vi "Handling calc param full_ext.vi"(0 "PV":dbl step=0.009999999776482582, 1 "SOURCE":u32=1 max=2 step=1, 2 "SOURCE_ALLOW":bool, 3 "PV2":dbl step=0.009999999776482582, 4 "control":T2={"GAIN"=1.0, "OFFSET"=0.0, "TIME_CONST"=100.0, "MINOFFSET"=2.0, "PVMIN"=0.0, "MINACC"=0.0, "LL"=1.0, "L"=2.0, "H"=8.0, "HH"=9.0, "MAXACC"=9.5, "PVMAX"=10.0, "MAXOFFSET"=2.0, "D"=0.5, "VMAX"=0.0, "TOUT"=1.0, "APERTURE"=0.0} {"APERTURE" min=-100000.0 max=100000.0 step=0.0010000000474974513; "TOUT" min=0.0 max=100000.0 step=1.0; "D" min=-100000.0 max=100000.0 step=0.0010000000474974513; "MAXOFFSET" min=0.0 max=50.0 step=0.0010000000474974513; "PVMAX" min=-100000.0 max=100000.0 step=0.0010000000474974513; "MAXACC" min=-100000.0 max=100000.0 step=0.0010000000474974513; "HH" min=-100000.0 max=100000.0 step=0.0010000000474974513; "H" min=-100000.0 max=100000.0 step=0.0010000000474974513; "L" min=-100000.0 max=100000.0 step=0.0010000000474974513; "LL" min=-100000.0 max=100000.0 step=0.0010000000474974513; "MINACC" min=-100000.0 max=100000.0 step=0.0010000000474974513; "PVMIN" min=-100000.0 max=100000.0 step=0.0010000000474974513; "MINOFFSET" min=0.0 max=50.0 step=0.0010000000474974513; "TIME_CONST" min=1.0 max=100000.0 step=1.0; "OFFSET" min=-100000.0 max=100000.0 step=0.0010000000474974513; "GAIN" min=0.0010000000474974513 max=1000.0 step=0.0010000000474974513}, 6 "initialise":bool, 7 "Sensor handling full reg old":T1, 8 "code":i32) -> (13 "Sensor handling full reg":T1, 14 "PVOUT":dbl format="%#_3g", 15 "SOURCEOUT":u32=1 max=2 step=1, 16 "STATE":T3, 17 "block":u32 format="%09b", 19 "ALRSTATE":errorcluster)   [LabVIEW 2019, in "Inputs.lvlib"]
uses:
  Inputs.lvlib
  Ctl/Parameter State.ctl
  Ctl/Sensor state.ctl
  Ctl/Sensor alarm.ctl
  Sensor_limit_Hd.vi
  Sensor_limit_Ld.vi
  Sensor_limit_H.vi
  Sensor_limit_L.vi
  Userlib.lvlib
  Trigers/Triggers.lvlib
panel:
  in  "UNIT":string
  in  "SENSOR":string
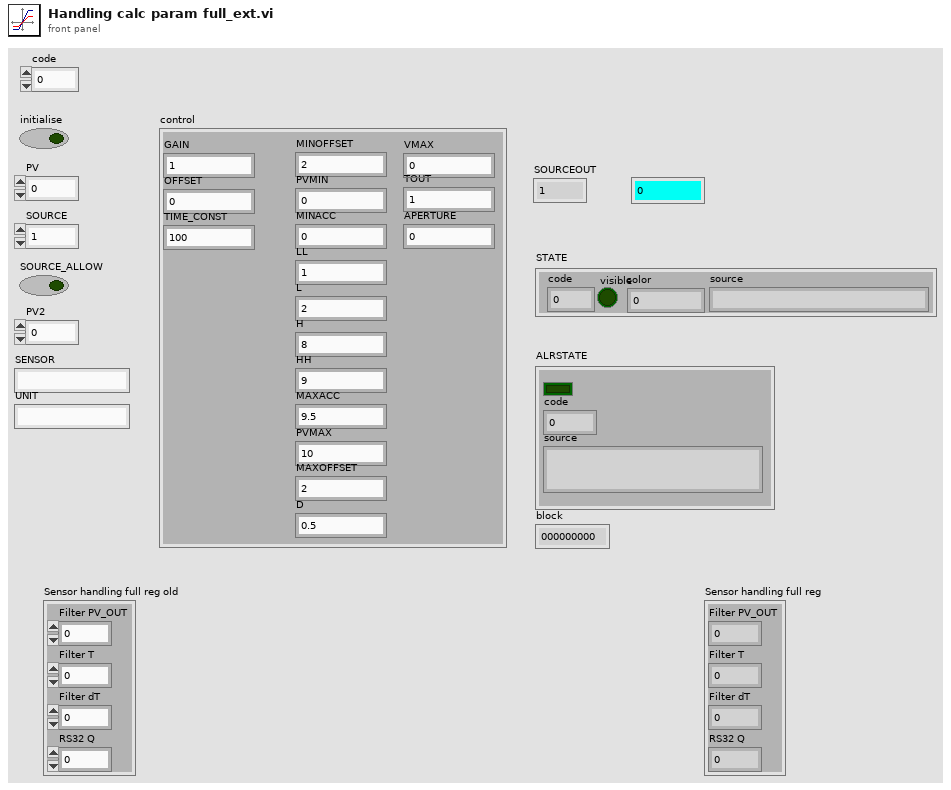
[diagram p1: front panel]
types:
  T1 = cluster{"Filter PV_OUT":dbl, "Filter T":dbl, "Filter dT":dbl, "RS32 Q":u32}
  T2 = cluster{"GAIN":dbl, "OFFSET":dbl, "TIME_CONST":dbl, "MINOFFSET":dbl, "PVMIN":dbl, "MINACC":dbl, "LL":dbl, "L":dbl, "H":dbl, "HH":dbl, "MAXACC":dbl, "PVMAX":dbl, "MAXOFFSET":dbl, "D":dbl, "VMAX":dbl, "TOUT":dbl, "APERTURE":dbl}
  T3 = typedef "Inputs.lvlib/Parameter State.ctl" = cluster{"code":i32, "visible":bool, "color":u32, "source":string}
  T4 = typedef "Inputs.lvlib/Sensor state.ctl" = cluster{"source":string, "color":u32, "visible":bool}[]
  T5 = typedef "Inputs.lvlib/Sensor alarm.ctl" = cluster{"source":string, "color":u32, "visible":bool}[]
  T6 = cluster{"source":string, "color":u32, "visible":bool}
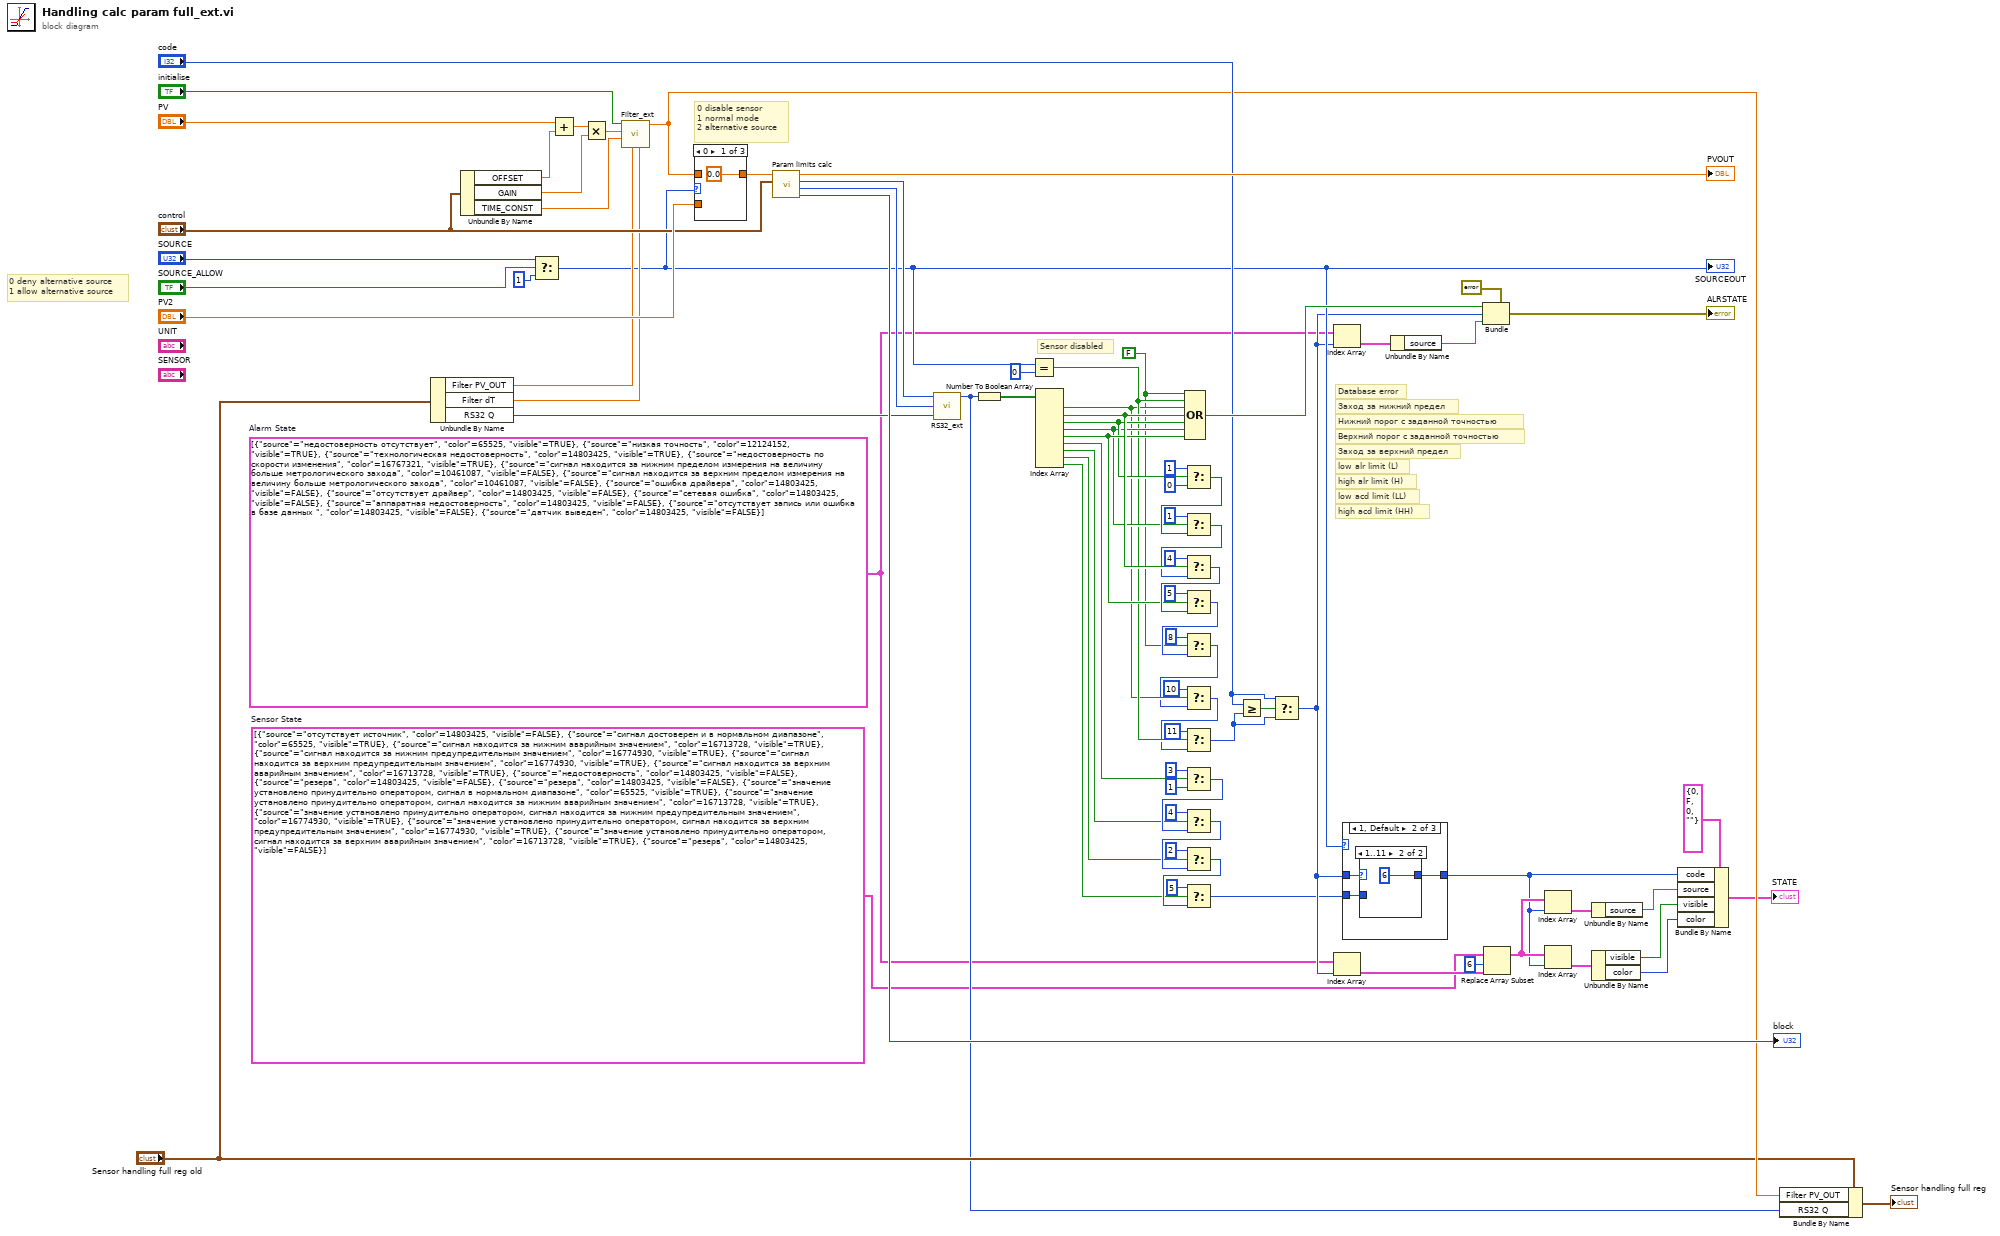
[diagram p0: block diagram]
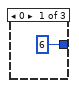
[diagram p2: hidden frame]
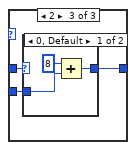
[diagram p4: hidden frame]
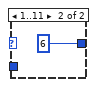
[diagram p5: hidden frame]
diagram:
  w1 = T4 [{"source"="отсутствует источник", "color"=14803425, "visible"=FALSE}, {"source"="сигнал достоверен и в нормальном диапазоне", "color"=65525, "visible"=TRUE}, {"source"="сигнал находится за нижним аварийным значением", "color"=16713728, "visible"=TRUE}, {"source"="сигнал находится за нижним предупредительным значением", "color"=16774930, "visible"=TRUE}, {"source"="сигнал находится за верхним предупредительным значением", "color"=16774930, "visible"=TRUE}, {"source"="сигнал находится за верхним аварийным значением", "color"=16713728, "visible"=TRUE}, {"source"="недостоверность", "color"=14803425, "visible"=FALSE}, {"source"="резерв", "color"=14803425, "visible"=FALSE}, {"source"="резерв", "color"=14803425, "visible"=FALSE}, {"source"="значение установлено принудительно оператором, сигнал в нормальном диапазоне", "color"=65525, "visible"=TRUE}, {"source"="значение установлено принудительно оператором, сигнал находится за нижним аварийным значением", "color"=16713728, "visible"=TRUE}, {"source"="значение установлено принудительно оператором, сигнал находится за нижним предупредительным значением", "color"=16774930, "visible"=TRUE}, {"source"="значение установлено принудительно оператором, сигнал находится за верхним предупредительным значением", "color"=16774930, "visible"=TRUE}, {"source"="значение установлено принудительно оператором, сигнал находится за верхним аварийным значением", "color"=16713728, "visible"=TRUE}, {"source"="резерв", "color"=14803425, "visible"=FALSE}]  # Sensor State
  w2 = T5 [{"source"="недостоверность отсутствует", "color"=65525, "visible"=TRUE}, {"source"="низкая точность", "color"=12124152, "visible"=TRUE}, {"source"="технологическая недостоверность", "color"=14803425, "visible"=TRUE}, {"source"="недостоверность по скорости изменения", "color"=16767321, "visible"=TRUE}, {"source"="сигнал находится за нижним пределом измерения на величину больше метрологического захода", "color"=10461087, "visible"=FALSE}, {"source"="сигнал находится за верхним пределом измерения на величину больше метрологического захода", "color"=10461087, "visible"=FALSE}, {"source"="ошибка драйвера", "color"=14803425, "visible"=FALSE}, {"source"="отсутствует драйвер", "color"=14803425, "visible"=FALSE}, {"source"="сетевая ошибка", "color"=14803425, "visible"=FALSE}, {"source"="аппаратная недостоверность", "color"=14803425, "visible"=FALSE}, {"source"="отсутствует запись или ошибка в базе данных ", "color"=14803425, "visible"=FALSE}, {"source"="датчик выведен", "color"=14803425, "visible"=FALSE}]  # Alarm State
  w26 = FALSE
  # "Database error"
  # "Верхний порог с заданной точностью"
  # "high acd limit (HH)"
  # "high alr limit (H)"
  # "low acd limit (LL)"
  # "low alr limit (L)"
  # "Заход за верхний предел"
  # "Нижний порог с заданной точностью"
  # "Заход за нижний предел"
  # "Sensor disabled"
  # "0 disable sensor\n1 normal mode\n2 alternative source"
  # "0 deny alternative source\n1 allow alternative source"
  n1 = Unbundle By Name("Sensor handling full reg old") -> ("Filter PV_OUT"=w22:dbl, "Filter dT"=w21:dbl, "RS32 Q"=w20:u32)
  n2 = Unbundle By Name("control") -> ("OFFSET"=w4:dbl, "GAIN"=w3:dbl, "TIME_CONST"=w30:dbl)
  n3 = Select(t="SOURCE", s="SOURCE_ALLOW", f=u32 1) -> (s? t:f=w11:u32)
  "SOURCEOUT" <- w11
  n4 = Add(x="PV", y=w4) -> (x+y=w7:dbl)
  n5 = Multiply(x=w7, y=w3) -> (x*y=w5:dbl)
  n6 = call "Filter_ext.vi"("dT"=w21, "PV_OUT old"=w22, "time_const ms"=w30, "PV"=w5, "Initialise"="initialise") -> ("PV_OUT"=w19:dbl)  [unwired: 6 in]
  n7 = case shown="0" w11 {
    tunnel: w19 -> [_ w85 _]
    tunnel: [0.0 w85 w86] -> w47
    tunnel: "PV2" -> [_ _ w86]
    frame 0 {
    }
    frame 1, Default {
    }
    frame 2 {
    }
  }
  n8 = call "Param limits calc.vi"("control"="control", "PV"=w47) -> ("block"=→"block":u32, "Off"=w45:u32, "On"=w46:u32, "PVOUT"=→"PVOUT":dbl)  [unwired: 2 in]
  n9 = call "RS32_ext.vi"("Q old"=w20, "R"=w45, "S"=w46) -> ("Q"=w12:u32)  [unwired: 1 in, 1 out]
  n10 = Number To Boolean Array(number=w12) -> (Boolean array=w65:bool[])
  n11 = Equal?(x=w11, y=u32 0) -> (x = y?=w50:bool)
  n12 = Index Array(array=w65) -> (element #1=w48:bool, element #2=w64:bool, element #3=w52:bool, element #4=w51:bool, element #5=w56:bool, element #6=w57:bool, element #7=w58:bool, element #8=w59:bool, element #9=w60:bool)  [unwired: 9 in]
  n13 = Compound Arithmetic op=OR ("status")(w26, w50, w48, w64, w52, w51, w56) -> (w69:bool)
  n14 = Select ("code")(t=1, s=w52, f=0) -> (s? t:f=w54:i32)
  n15 = Select ("code")(t=1, s=w51, f=w54) -> (s? t:f=w53:i32)
  n16 = Select ("code")(t=4, s=w64, f=w53) -> (s? t:f=w78:i32)
  n17 = Select ("code")(t=5, s=w56, f=w78) -> (s? t:f=w33:i32)
  n18 = Select ("code")(t=8, s=w26, f=w33) -> (s? t:f=w32:i32)
  n19 = Select ("code")(t=10, s=w48, f=w32) -> (s? t:f=w37:i32)
  n20 = Select ("code")(t=11, s=w50, f=w37) -> (s? t:f=w24:i32)
  n21 = Select ("code")(t=3 ("code"), s=w57, f=1 ("code")) -> (s? t:f=w73:i32)
  n22 = Select ("code")(t=4 ("code"), s=w58, f=w73) -> (s? t:f=w72:i32)
  n23 = Select ("code")(t=2 ("code"), s=w59, f=w72) -> (s? t:f=w70:i32)
  n24 = Select ("code")(t=5 ("code"), s=w60, f=w70) -> (s? t:f=w9:i32)
  n25 = Greater Or Equal?(x="code", y=w24) -> (x >= y?=w25:bool)
  n26 = Select(t="code", s=w25, f=w24) -> (s? t:f=w10:i32)
  n27 = Index Array(array=w2, index=w10) -> (element=w41:T6)
  n28 = Index Array(array=w2, index=w10) -> (element=w40:T6)
  n29 = case "code" shown="1, Default" w11 {
    tunnel: w10 -> [_ w90 w95]
    tunnel: w9 -> [_ w89 w94]
    tunnel: [6 ("code") w88 w93] -> w8
    frame 0 {
    }
    frame 1, Default {
      n30 = case "code" shown="1..11" w90 {
        tunnel: [w91 6 ("code")] -> w88
        tunnel: w89 -> [w91 _]
        frame 0, Default {
        }
        frame 1..11 {
        }
      }
    }
    frame 2 {
      n31 = case "code" shown="0, Default" w95 {
        tunnel: [w97 6 ("code")] -> w93
        tunnel: w94 -> [w98 _]
        frame 0, Default {
          n32 = Add ("code")(x=8 ("code"), y=w98) -> (x+y=w97:i32)
        }
        frame 1..11 {
        }
      }
    }
  }
  n33 = Unbundle By Name(w41) -> ("source"=w42:string)
  n34 = Bundle(cluster=cluster{bool, i32, "source":string} {FALSE, 0, "source"=""}, w69, w10, "source"=w42) -> (→"ALRSTATE":cluster{bool, i32, "source":string})
  n35 = Replace Array Subset(array=w1, new element=w40, index=6) -> (w13:T4)
  n36 = Index Array(array=w13, index=w8) -> (element=w36:T6)
  n37 = Index Array(array=w13, index=w8) -> (element=w38:T6)
  n38 = Unbundle By Name(w36) -> ("source"=w39:string)
  n39 = Unbundle By Name(w38) -> ("visible"=w35:bool, "color"=w31:u32)
  n40 = Bundle By Name(cluster=T3 {"code"=0, "visible"=FALSE, "color"=0, "source"=""} ("STATE"), "code"=w8, "source"=w39, "visible"=w35, "color"=w31) -> (→"STATE":T3)
  n41 = Bundle By Name(cluster="Sensor handling full reg old", "Filter PV_OUT"=w19, "RS32 Q"=w12) -> (→"Sensor handling full reg":T1)
